vi "Generate Command String.vi"(0 "ITX Commands in":refnum<class "ITX Commands.lvclass">, 1 "ITX Commands in":string, 3 "error in (no error)":errorcluster) -> (7 "ITX Commands out":refnum<class "ITX Commands.lvclass">, 8 "ITX Commands":string, 10 "error out":errorcluster)   [LabVIEW 2019, in "ITX Commands.lvclass"]
uses:
  ITX Commands.lvclass
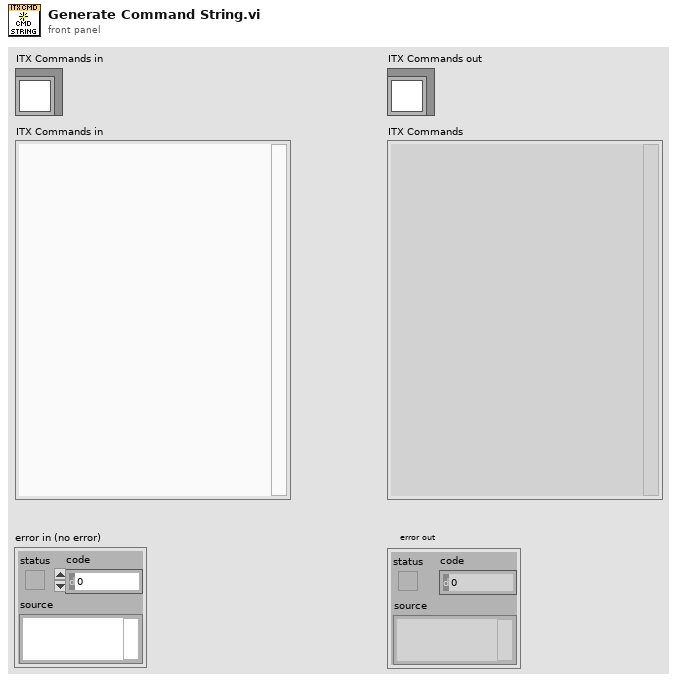
[diagram p1: front panel]
types:
  T1 = cluster{"axThick":string, "grid":string, "height":string, "Log":string, "mirror":string, "prescaleExp":string, "rgb":string, "width":string}
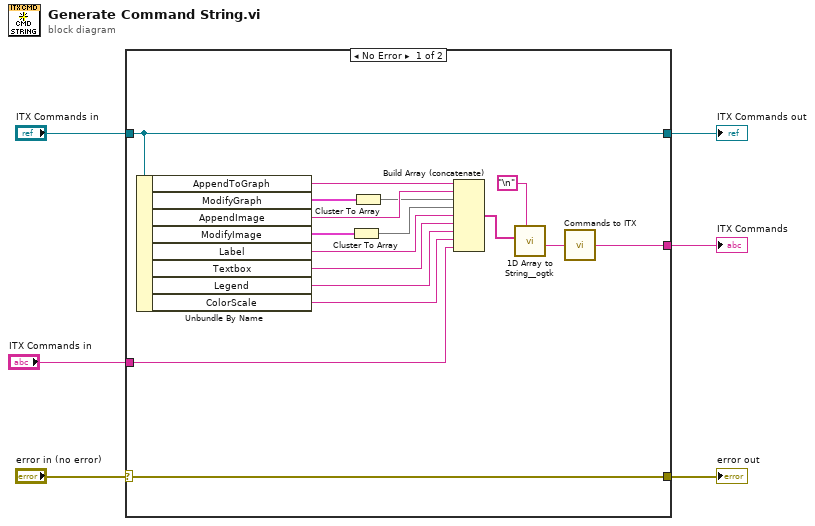
[diagram p0: block diagram]
diagram:
  n1 = case shown="No Error" "error in (no error)" {
    selector: "error in (no error)" -> [w23 w25]
    tunnel: [w23 w25] -> w5
    tunnel: [w19 w24] -> w3
    tunnel: "ITX Commands in" -> [w19 w24]
    tunnel: [w20 _] -> w2
    tunnel: "ITX Commands in" -> [w9 _]
    frame No Error {
      n2 = Unbundle By Name(w19) -> ("AppendToGraph"=w16:string, "ModifyGraph"=w18:T1, "AppendImage"=w8:string, "ModifyImage"=w17:cluster{"ctab":string}, "Label"=w14:string, "Textbox"=w13:string, "Legend"=w12:string, "ColorScale"=w10:string)
      n3 = Cluster To Array(cluster=w17) -> (array=w15:string[])
      n4 = Cluster To Array(cluster=w18) -> (array=w7:string[])
      n5 = Build Array (concatenate)(w16, w8, w7, w15, w14, w13, w12, w10, w9) -> (w11:string[])
      n6 = call "1D Array to String__ogtk.vi"("delimiter (Tab)"="\n", "Array of Strings"=w11) -> ("delimited string"=w21:string)  [unwired: 9 in]
      n7 = call "Commands to ITX.vi"("Commands"=w21) -> ("ITX Commands"=w20:string)
    }
    frame Error {
    }
  }
  "error out" <- w5
  "ITX Commands out" <- w3
  "ITX Commands" <- w2
